vi "Run Server.vi"(8 "error in (no error)":errorcluster, 11 "Stop OOB Server UE":refnum<user-event>) -> (0 "error out":errorcluster)   [LabVIEW 2025, in "OOB gRPC Server.lvlib"]
uses:
  OOB gRPC Server.lvlib
  <vilib>/gRPC/LabVIEW gRPC Servicer/ServiceBase/ServiceBase.lvclass
  <vilib>/gRPC/LabVIEW gRPC Servicer/Servicer/Servicer.lvclass
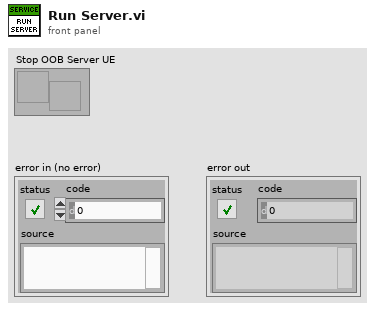
[diagram p1: front panel]
types:
  T1 = enum32{"Invalid", "Standard", "Closed", "Hidden", "Minimized", "Maximized"}
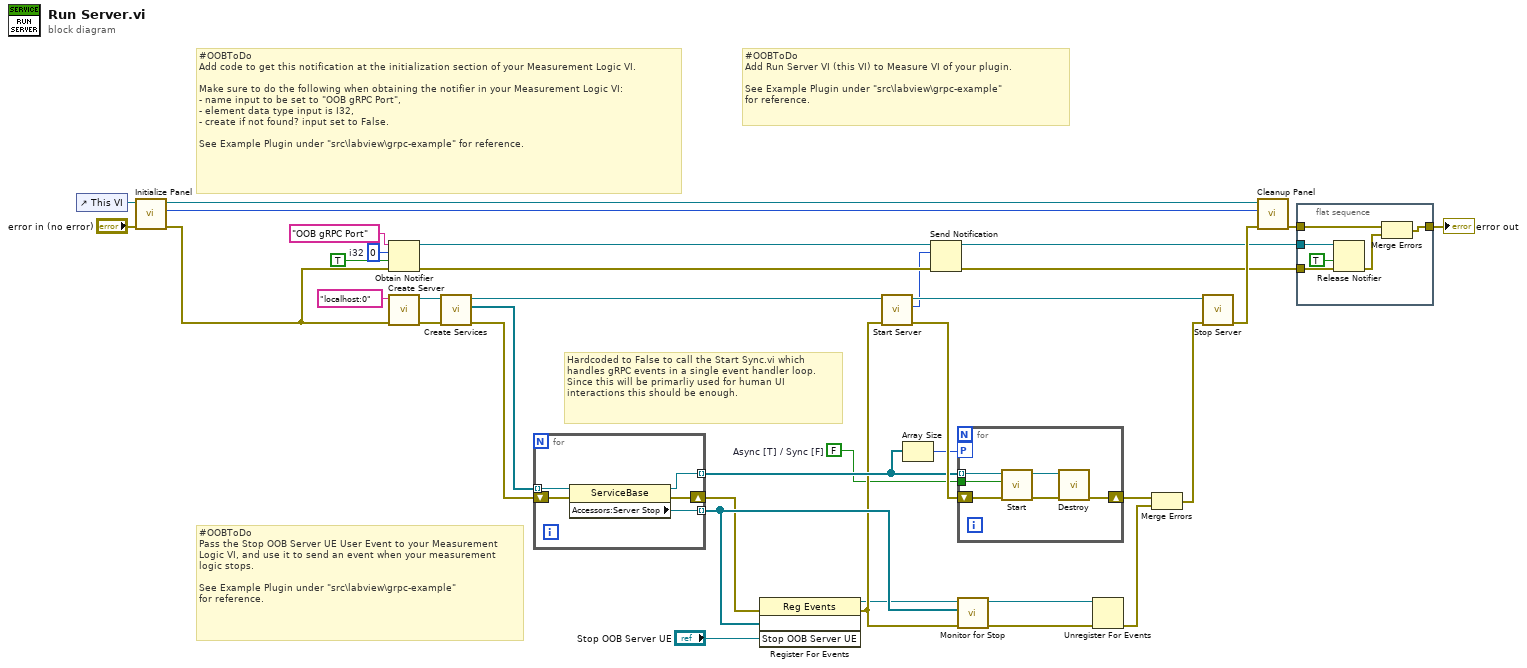
[diagram p0: block diagram]
diagram:
  w2 = FALSE  # Async [T] / Sync [F]
  w11 = 0  # i32
  # "#OOBToDo \nPass the Stop OOB Server UE User Event to your Measurement Logic VI, and use it to send an event when your measurement logic stops.\n\nSee Example Plugin under \"src\\labview\\grpc-example\" for reference."
  # "#OOBToDo \nAdd Run Server VI (this VI) to Measure VI of your plugin.\n\nSee Example Plugin under \"src\\labview\\grpc-example\" for reference."
  # "Hardcoded to False to call the Start Sync.vi which handles gRPC events in a single event handler loop.\nSince this will be primarliy used for human UI interactions this should be enough."
  # "#OOBToDo \nAdd code to get this notification at the initialization section of your Measurement Logic VI. \n\nMake sure to do the following when obtaining the notifier in your Measurement Logic VI:\n- name input to be set to \"OOB gRPC Port\",\n- element data type input is I32,\n- create if not found? input set to False.\n\nSee Example Plugin under \"src\\labview\\grpc-example\" for reference."
  n1 = control-ref of="This VI"() -> (w23:refnum<vi>)
  n2 = call "Initialize Panel.vi"("error in (no error)"="error in (no error)", "vi reference in"=w23) -> ("error out"=w6:errorcluster, "initial window state"=w21:T1, "vi reference out"=w22:refnum<vi>)  [unwired: 7 in]
  n3 = Obtain Notifier(name (unnamed)="OOB gRPC Port", notification data type=w11, create if not found? (T)=TRUE, error in (no error)=w6) -> (notifier out=w9:refnum<notifier>, error out=w8:errorcluster)  [unwired: 1 out]
  n4 = call <vilib>:"Create Server.vi"("error in"=w6, "Server Address"="localhost:0") -> ("error out"=w19:errorcluster, "gRPC server out"=w36:refnum<class "Servicer.lvclass">)  [unwired: 8 in]
  n5 = call "Create Services.vi"("error in (no error)"=w19, "gRPC server in"=w36) -> ("error out"=w18:errorcluster, "gRPC services out"=w17:refnum<class "ServiceBase.lvclass">[], "gRPC server out"=w35:refnum<class "Servicer.lvclass">)  [unwired: 7 in]
  n6 = for {
    tunnel: [w41] -> w31 mode=indexing
    shift-right: [w40] -> w30
    shift-left: w18 -> [w38]
    tunnel: [w42] -> w32 mode=indexing
    tunnel: w17 -> [w39] mode=indexing
    n7 = property class="ServiceBase"(reference=w39, error in=w38) -> (reference out=w42:refnum<class "ServiceBase.lvclass">, error out=w40:errorcluster, "Accessors:Server Stop"=w41:refnum<user-event>)
  }
  n8 = register-events(error in=w30, w31, "Stop OOB Server UE") -> (reference out=w1:refnum<event-registration>, error out=w29:errorcluster)  [unwired: 1 in]
  n9 = call <vilib>:"Start Server.vi"("error in"=w29, "gRPC server in"=w35) -> ("error out"=w34:errorcluster, "Listening Port"=w5:i32, "gRPC server out"=w37:refnum<class "Servicer.lvclass">)  [unwired: 7 in]
  n10 = Array Size(array=w32) -> (size(s)=w33:i32)
  n11 = Send Notification(notification=w5, notifier=w9, error in (no error)=w8) -> (notifier out=w4:refnum<notifier>, error out=w3:errorcluster)
  n12 = for {
    tunnel: w32 -> [w46] mode=indexing
    tunnel: w2 -> [w44]
    workers-P: w33 -> [_]
    shift-right: [w43] -> w28
    shift-left: w34 -> [w45]
    n13 = call-dynamic "Start.vi"("error in"=w45, "ASync [T]"=w44, "gRPC service in"=w46) -> ("error out"=w47:errorcluster, "gRPC service out"=w48:refnum<class "ServiceBase.lvclass">)  [unwired: 7 in]
    n14 = call-dynamic "Destroy.vi"("error in"=w47, "gRPC service in"=w48) -> ("error out"=w43:errorcluster)  [unwired: 8 in, 1 out]
  }
  n15 = call "Monitor for Stop.vi"("error in (no error)"=w29, "service stop events"=w31, "Event Registration Refnum in"=w1) -> ("error out"=w24:errorcluster, "Event Registration Refnum out"=w26:refnum<event-registration>)  [unwired: 7 in]
  n16 = Unregister For Events(event registration refnum=w26, error in=w24) -> (error out=w25:errorcluster)
  n17 = Merge Errors(w28, w25) -> (w27:errorcluster)
  n18 = call <vilib>:"Stop Server.vi"("error in"=w27, "gRPC server in"=w37) -> ("error out"=w20:errorcluster)  [unwired: 9 in]
  n19 = call "Cleanup Panel.vi"("error in (no error)"=w20, "initial window state"=w21, "vi reference in"=w22) -> ("error out"=w14:errorcluster)  [unwired: 7 in, 1 out]
  n20 = flat-sequence {
    tunnel: w4 -> [w54]
    tunnel: w14 -> [w52]
    tunnel: [w51] -> w13
    tunnel: w3 -> [w49]
    frame #0 {
      n21 = Release Notifier(notifier=w54, force destroy? (F)=TRUE, error in (no error)=w49) -> (error out=w50:errorcluster)  [unwired: 2 out]
      n22 = Merge Errors(w52, w50) -> (w51:errorcluster)
    }
  }
  "error out" <- w13
